vi "Write PacMan Arc.vi"(8 "error in (no error)":errorcluster, 10 "PacMan Arc":T1, 11 "PacMan in":refnum<class "PacMan.lvclass">) -> (0 "error out":errorcluster, 3 "PacMan out":refnum<class "PacMan.lvclass">)   [LabVIEW 2016, in "PacManClasses.lvlib" / "PacMan.lvclass"]
uses:
  PacMan.lvclass
  Generic Controls/PacMan Arc.ctl
  PacMan.lvclass/PacMan.ctl
  PacManClasses.lvlib
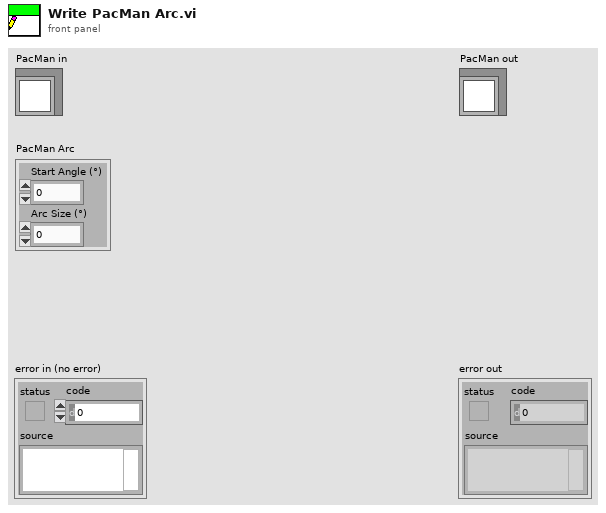
[diagram p1: front panel]
types:
  T1 = typedef "PacManClasses.lvlib/PacMan Arc.ctl" = cluster{"Start Angle (°)":i16, "Arc Size (°)":i16}
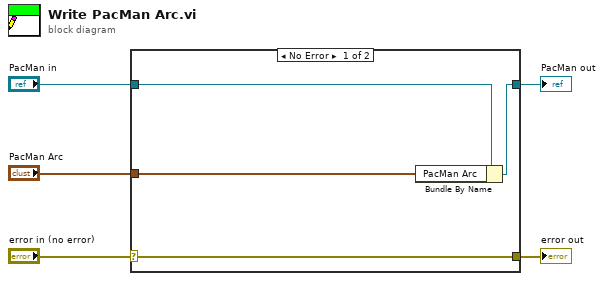
[diagram p0: block diagram]
diagram:
  n1 = case shown="No Error" "error in (no error)" {
    selector: "error in (no error)" -> [w9 w10]
    tunnel: [w9 w10] -> w4
    tunnel: [w7 w11] -> w2
    tunnel: "PacMan in" -> [w8 w11]
    tunnel: "PacMan Arc" -> [w6 _]
    frame No Error {
      n2 = Bundle By Name(cluster=w8, "PacMan Arc"=w6) -> (w7:refnum<class "PacMan.lvclass">)
    }
    frame Error {
    }
  }
  "error out" <- w4
  "PacMan out" <- w2
